vi "LPF_comparison.vi"() -> ()   [LabVIEW 2020]
uses:
  <vilib>/express/express analysis/Spectral/Block/exnSpectralBlock spectral measurements peak poly.vi
  <vilib>/express/express analysis/Spectral/Block/exnSpectralBlock spectral measurements peak DDT.vi
  <vilib>/express/express analysis/Spectral/XNode/ExpressSpectralMeasurementsBlockNode.xnode
panel:
  out "Waveform":dbl[][](graph)
  out "FFT Spectrum":dbl[][](graph)
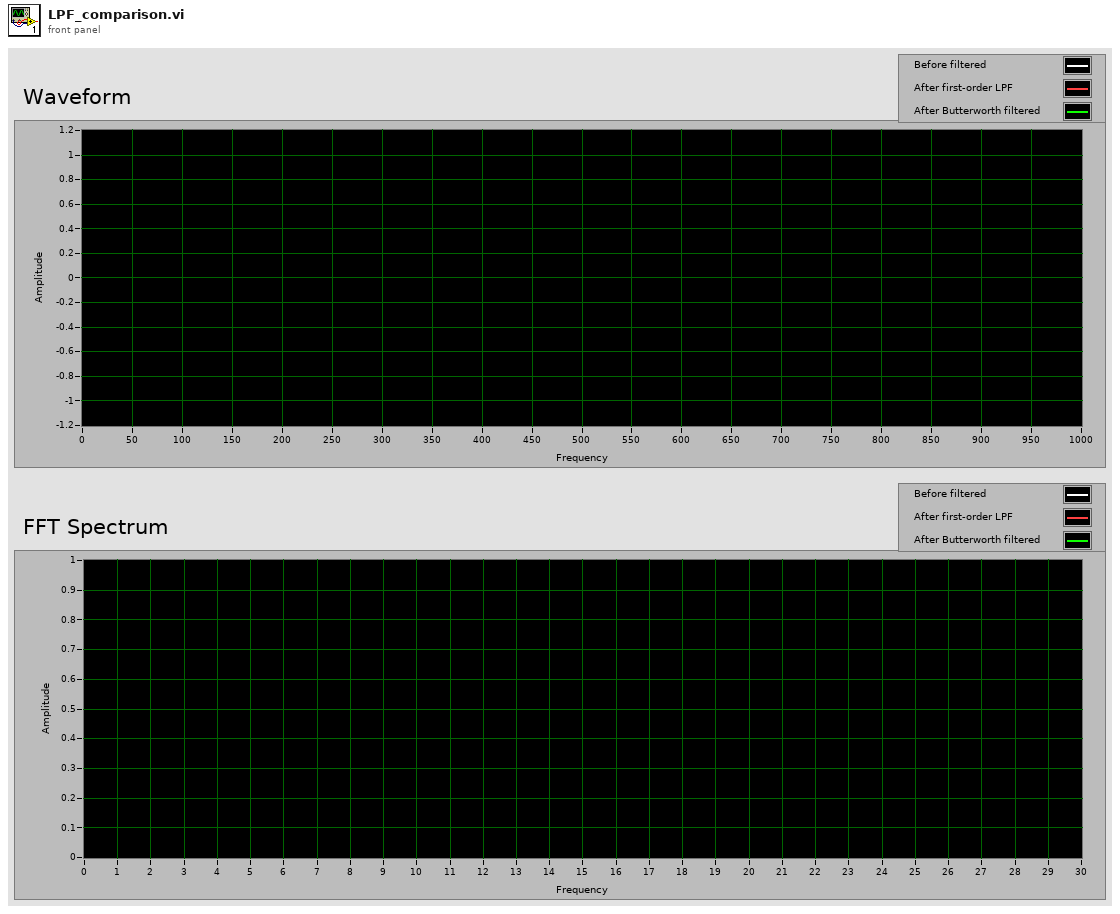
[diagram p1: front panel]
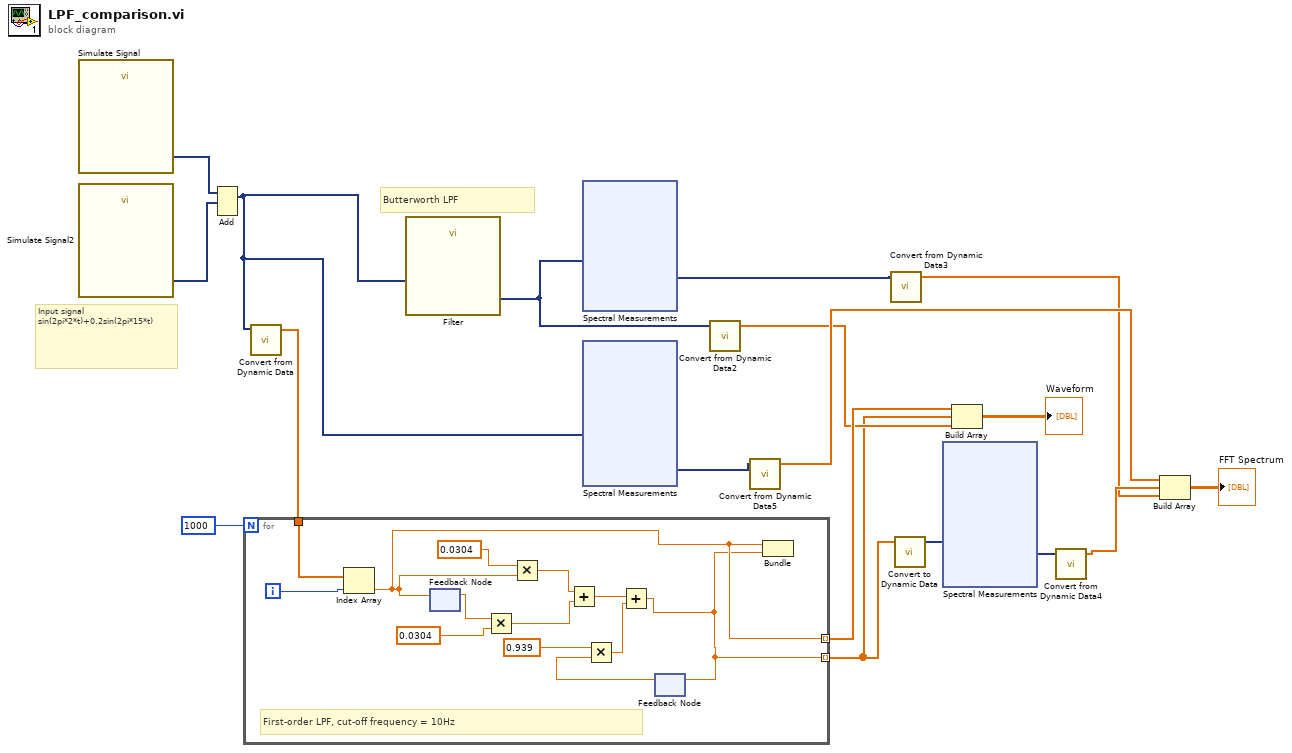
[diagram p0: block diagram]
diagram:
  # "Input signal\nsin(2pi*2*t)+0.2sin(2pi*15*t)"
  # "Butterworth LPF"
  n1 = call "Simulate Signal"() -> ("Sine"=w18:dynamicdata)  [unwired: 14 in, 1 out]
  n2 = call "Simulate Signal2"() -> ("Sine"=w17:dynamicdata)  [unwired: 14 in, 1 out]
  n3 = Add(1:w17, 2:w18) -> (0:w8:dynamicdata)  [unwired: 1 in, 1 out]
  n4 = call "Convert from Dynamic Data"("Dynamic Data Type"=w8) -> ("Array"=w15:dbl[])  [unwired: 3 in]
  n5 = for {
    N: 1000 -> [_]
    tunnel: w15 -> [w22]
    tunnel: [w20] -> w5 mode=indexing
    tunnel: [w19] -> w3 mode=indexing
    i -> [w21]
    # "First-order LPF, cut-off frequency = 10Hz"
    n6 = Index Array(array=w22, index=w21) -> (element=w20:dbl)
    n7 = feedback #1() -> (w31:dbl)  [unwired: 1 in]
    n8 = feedback-in #1(w20) -> ()
    n9 = Multiply(x=w31, y=0.0304) -> (x*y=w27:dbl)
    n10 = Multiply(x=0.0304, y=w20) -> (x*y=w28:dbl)
    n11 = Add(x=w28, y=w27) -> (x+y=w26:dbl)
    n12 = feedback #2() -> (w25:dbl)  [unwired: 1 in]
    n13 = Multiply(x=0.939, y=w25) -> (x*y=w23:dbl)
    n14 = Add(x=w26, y=w23) -> (x+y=w19:dbl)
    n15 = feedback-in #2(w19) -> ()
    n16 = Bundle(w20, w19) -> ()  [unwired: 1 in, 1 out]
  }
  n17 = call "Filter"("Signal"=w8) -> ("Filtered Signal"=w14:dynamicdata)  [unwired: 9 in, 1 out]
  n18 = xnode "Spectral Measurements"("Signals"=w14) -> ("FFT - (Peak)"=w11:dynamicdata)  [unwired: 1 in, 2 out]
  n19 = xnode "Spectral Measurements"("Signals"=w8) -> ("FFT - (Peak)"=w7:dynamicdata)  [unwired: 1 in, 2 out]
  n20 = call "Convert from Dynamic Data2"("Dynamic Data Type"=w14) -> ("Array"=w4:dbl[])  [unwired: 3 in]
  n21 = call "Convert from Dynamic Data5"("Dynamic Data Type"=w7) -> ("Array"=w6:dbl[])  [unwired: 3 in]
  n22 = call "Convert from Dynamic Data3"("Dynamic Data Type"=w11) -> ("Array"=w1:dbl[])  [unwired: 3 in]
  n23 = call "Convert to Dynamic Data"("Array"=w3) -> ("Dynamic Data Type"=w12:dynamicdata)  [unwired: 3 in]
  n24 = xnode "Spectral Measurements"("Signals"=w12) -> ("FFT - (Peak)"=w10:dynamicdata)  [unwired: 1 in, 2 out]
  n25 = Build Array(w5, w3, w4) -> (→"Waveform":dbl[][])
  n26 = call "Convert from Dynamic Data4"("Dynamic Data Type"=w10) -> ("Array"=w2:dbl[])  [unwired: 3 in]
  n27 = Build Array(w6, w2, w1) -> (→"FFT Spectrum":dbl[][])
